vi "ModeArray.vi"(1 "Write Array":u16[](array[numeric]), 2 "Write?":bool) -> (0 "Array":u16[](array[numeric]))   [LabVIEW 2012, in "FTC.lvlib" / "Remote Interface.lvlib"]
uses:
  Remote Interface.lvlib
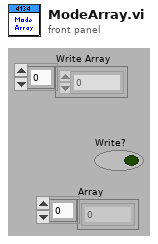
[diagram p1: front panel]
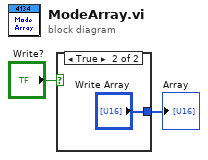
[diagram p0: block diagram]
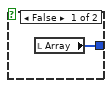
[diagram p2: hidden frame]
diagram:
  n1 = case shown="True" "Write?" {
    tunnel: [w3 "Write Array"] -> w1
    frame False {
      n2 = local read "Array"() -> (w3:u16[])
    }
    frame True {
    }
  }
  "Array" <- w1
